vi "Calculate Refactor Metrics for Project.vi"(8 "error in":errorcluster, 9 "refactored dependencies":T3(array[cluster]), 10 "refactored classes":path[](array[path]), 11 "project path":path) -> (0 "error out":errorcluster, 3 "refactor results":T2)   [LabVIEW 2020, in "MeasurementService Editor.lvlib"]
uses:
  MeasurementService Editor.lvlib
  Rename Refactor Result.ctl
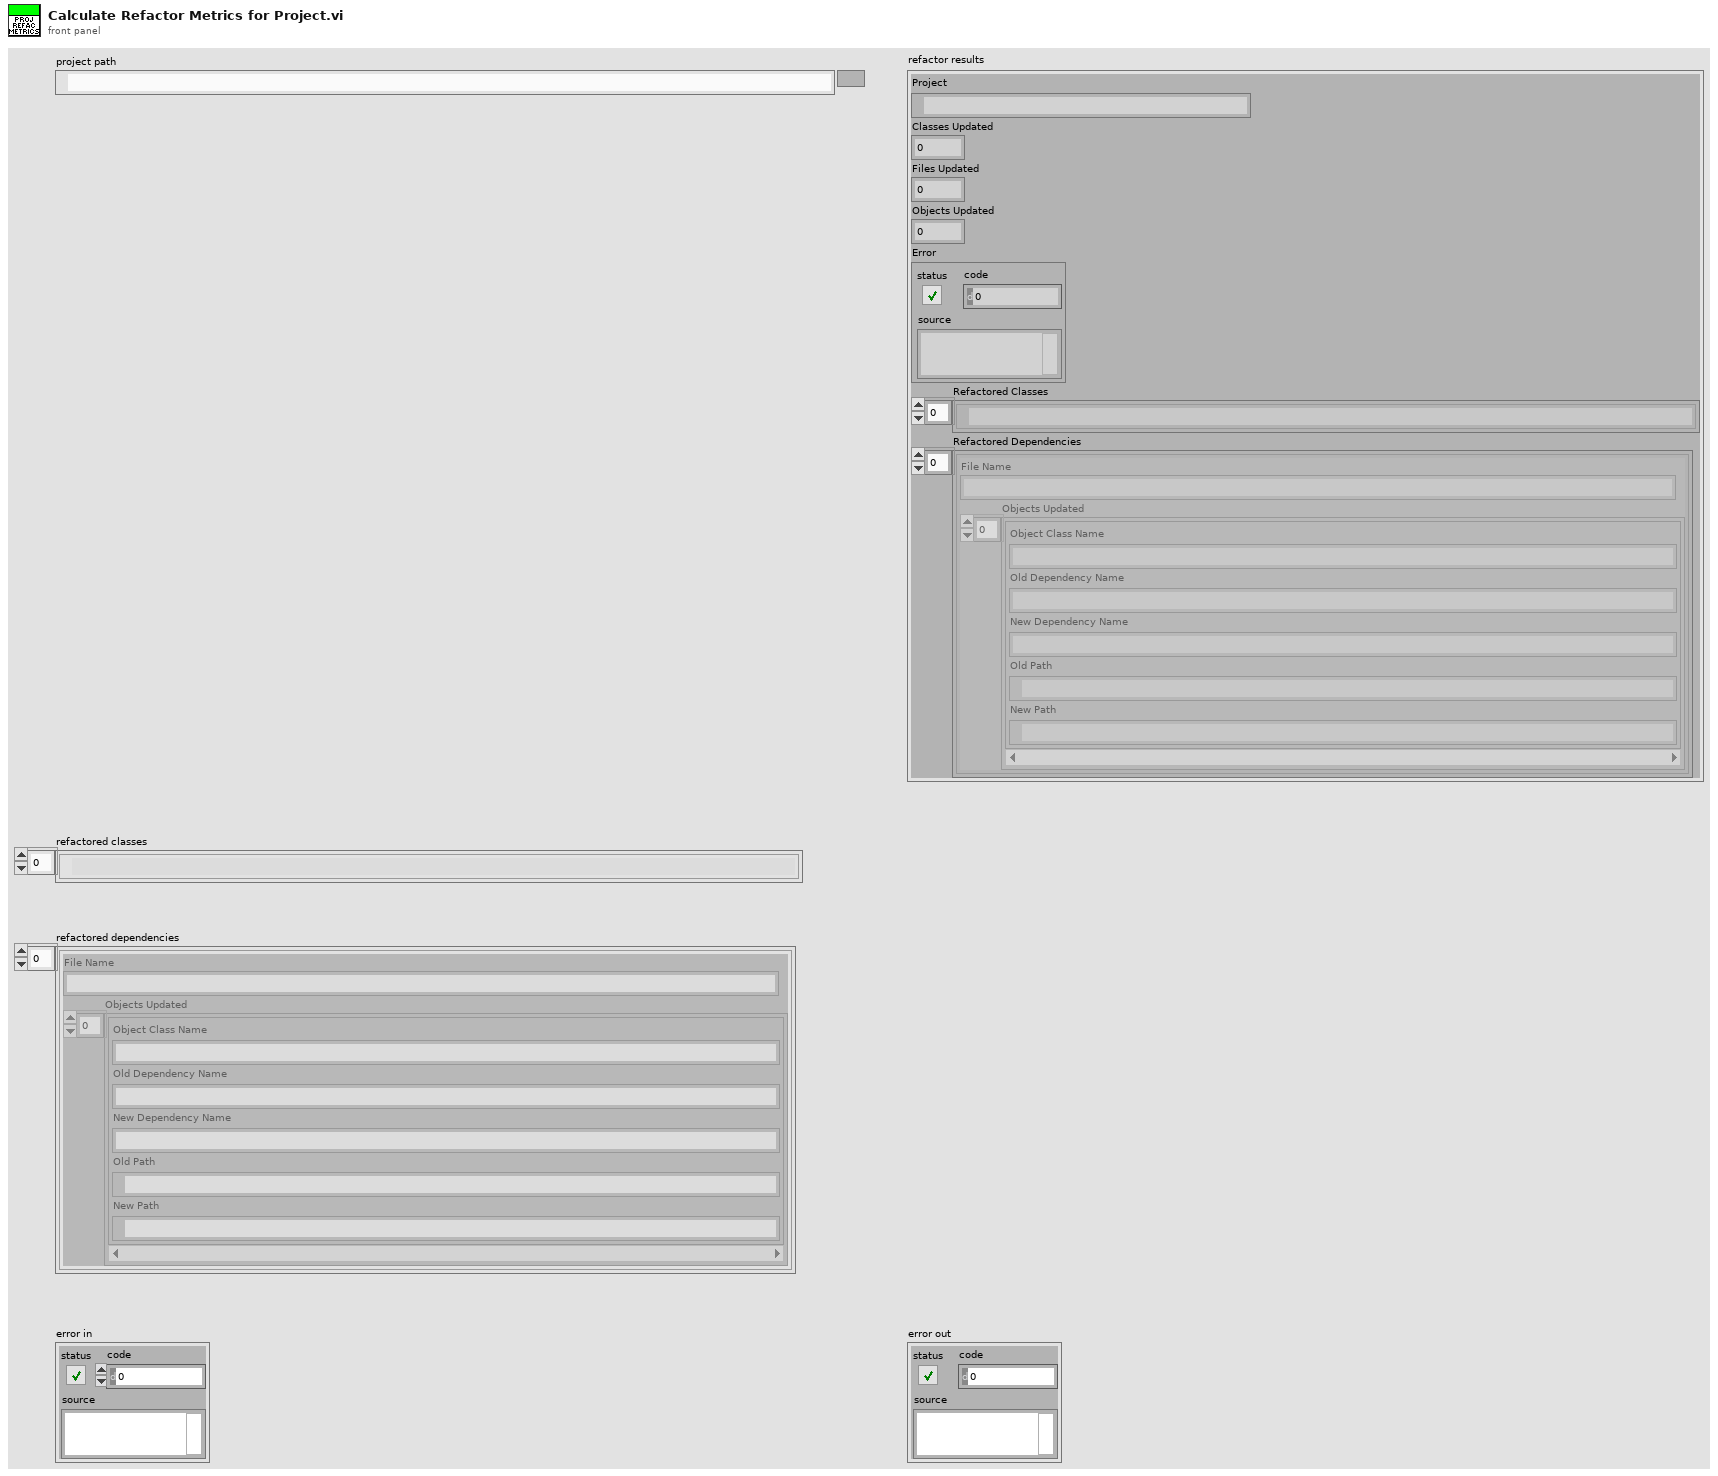
[diagram p1: front panel]
types:
  T1 = typedef "MeasurementService Editor.lvlib/Rename Refactor Result.ctl" = cluster{"Object Class Name":string, "Old Dependency Name":string, "New Dependency Name":string, "Old Path":path, "New Path":path}
  T2 = cluster{"Project":path, "Classes Updated":u32, "Files Updated":u32, "Objects Updated":u32, "Error":errorcluster, "Refactored Classes":path[], "Refactored Dependencies":cluster{"File Name":string, "Objects Updated":T1[]}[]}
  T3 = cluster{"File Name":string, "Objects Updated":T1[]}[]
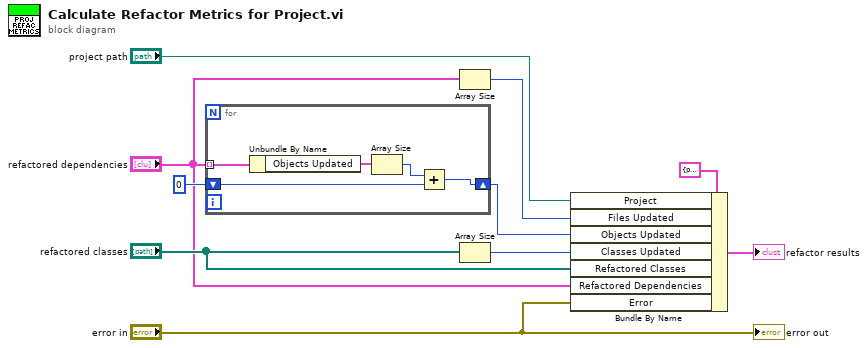
[diagram p0: block diagram]
diagram:
  n1 = for {
    tunnel: "refactored dependencies" -> [w15] mode=indexing
    shift-right: [w11] -> w3
    shift-left: 0 -> [w12]
    n2 = Unbundle By Name(w15) -> ("Objects Updated"=w14:T1[])
    n3 = Array Size(array=w14) -> (size(s)=w13:i32)
    n4 = Add(x=w13, y=w12) -> (x+y=w11:i32)
  }
  n5 = Array Size(array="refactored dependencies") -> (size(s)=w2:i32)
  n6 = Array Size(array="refactored classes") -> (size(s)=w4:i32)
  n7 = Bundle By Name(cluster=T2 {"Project"=path "", "Classes Updated"=0, "Files Updated"=0, "Objects Updated"=0, "Error"={"status"=FALSE, "code"=0, "source"=""}, "Refactored Classes"=[], "Refactored Dependencies"=[]} ("refactor results"), "Project"="project path", "Files Updated"=w2, "Objects Updated"=w3, "Classes Updated"=w4, "Refactored Classes"="refactored classes", "Refactored Dependencies"="refactored dependencies", "Error"="error in") -> (→"refactor results":T2)
  "error out" <- "error in"
